vi "subVIContent.vi"   [LabVIEW 2018]
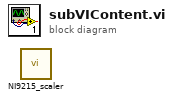
[diagram p0: block diagram]
diagram:
  n1 = call "NI9215_scaler.vi"() -> ()  [unwired: 12 in]
